vi "Rbf_kernel.vi"(8 "error in":errorcluster caption="entrée d'erreur", 9 "Y":string[][](array[string]), 10 "X":string[][](array[string]), 11 "rbf_kernel":cluster{"gamma":string}={"gamma"="None"}) -> (0 "error out":errorcluster caption="sortie d'erreur", 3 "Data":T1)   [LabVIEW 2020]
doc: "Compute the rbf (gaussian) kernel between X and Y:\n\nK(x, y) = exp(-gamma ||x-y||^2)\n\nfor each pair of rows x in X and y in Y.\n\nParameters : \n\n- X : array of shape (n_samples_X, n_features)\n\n- Y : array of shape (n_samples_Y, n_features)\n\n- gamma : float, default None\nIf None, defaults to 1.0 / n_features\n\nReturns : \n\n- kernel_matrix : array of shape (n_samples_X, n_samples_Y)"
uses:
  Rbf_kernel.lvclass
panel:
  out "Rbf_kernel.lvclass":refnum<class "Rbf_kernel.lvclass">
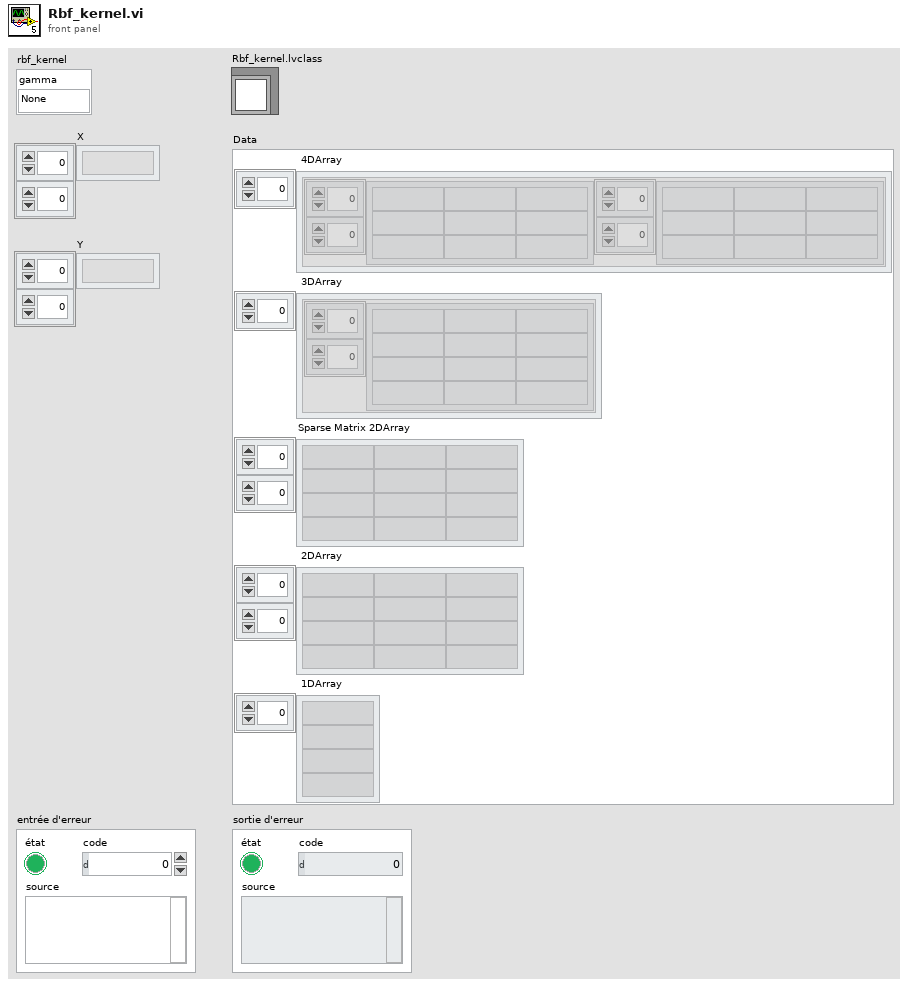
[diagram p1: front panel]
types:
  T1 = cluster{" 4DArray":cluster{"1":string[][], "2":string[][]}[], " 3DArray":cluster{"Tableau":string[][]}[], "Sparse Matrix 2DArray":string[][], " 2DArray":string[][], " 1DArray":string[]}
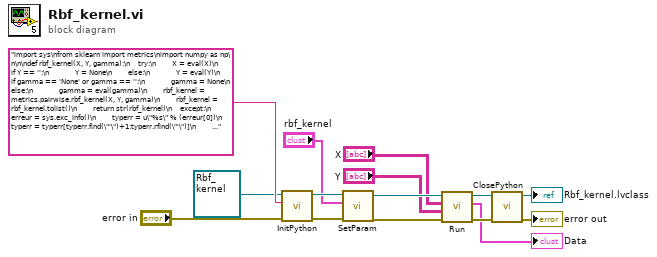
[diagram p0: block diagram]
diagram:
  n1 = call-dynamic "InitPython.vi"("error in (no error)"="error in", "Python Instruction"="import sys\nfrom sklearn import metrics\nimport numpy as np\n\n\ndef rbf_kernel(X, Y, gamma):\n    try:\n        X = eval(X)\n        if Y == '':\n             Y = None\n        else:\n             Y = eval(Y)\n        if gamma == 'None' or gamma == '':\n             gamma = None\n        else:\n             gamma = eval(gamma)\n        rbf_kernel = metrics.pairwise.rbf_kernel(X, Y, gamma)\n        rbf_kernel = rbf_kernel.tolist()\n        return str(rbf_kernel)\n    except:\n        erreur = sys.exc_info()\n        typerr = u\"%s\" % (erreur[0])\n        typerr = typerr[typerr.find(\"'\")+1:typerr.rfind(\"'\")]\n        msgerr = u\"%s\" % (erreur[1])\n        message = str('/!\\\\ {0} : {1}'. format(typerr,msgerr))\n        return message", "Scikit-learn en entrée"=refnum<class "Rbf_kernel.lvclass"> refnum ("Rbf_kernel.lvclass")) -> ("error out"=w11:errorcluster, "Scikit-learn en sortie"=w12:refnum<class "Rbf_kernel.lvclass">)  [unwired: 7 in]
  n2 = call-dynamic "SetParam.vi"("error in (no error)"=w11, "rbf_kernel"="rbf_kernel", "Rbf_kernel.lvclass"=w12) -> ("error out"=w7:errorcluster, "Rbf_kernel.lvclass"=w8:refnum<class "Rbf_kernel.lvclass">)  [unwired: 7 in]
  n3 = call-dynamic "Run.vi"("error in (no error)"=w7, "Y"="Y", "X"="X", "Rbf_kernel.lvclass"=w8) -> ("error out"=w9:errorcluster, "Data"=→"Data":T1, "Rbf_kernel.lvclass"=w10:refnum<class "Rbf_kernel.lvclass">)  [unwired: 5 in]
  n4 = call-dynamic "ClosePython.vi"("error in (no error)"=w9, "Scikit-learn en entrée"=w10) -> ("error out"=→"error out":errorcluster, "Scikit-learn en sortie"=→"Rbf_kernel.lvclass":refnum<class "Rbf_kernel.lvclass">)  [unwired: 8 in]
